vi "Count_Hardness_test.vi"(0 "HS":sgl[](array[numeric]), 1 "TV":sgl[][](array[numeric])) -> (2 "AVG":sgl[](array[numeric]), 3 "HV":sgl[](array[numeric]) format="%#.2g", 4 "REP":sgl[](array[numeric]) format="%#.2g")   [LabVIEW 2019]
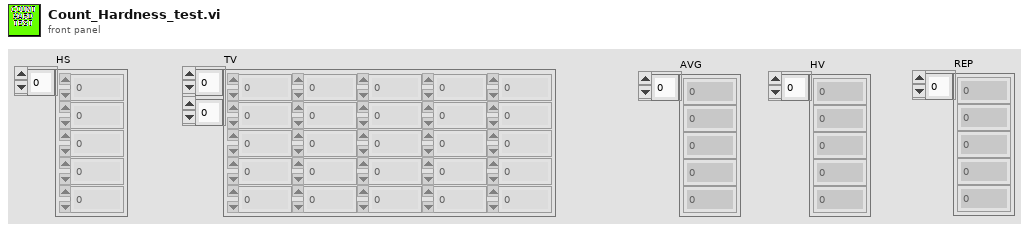
[diagram p1: front panel]
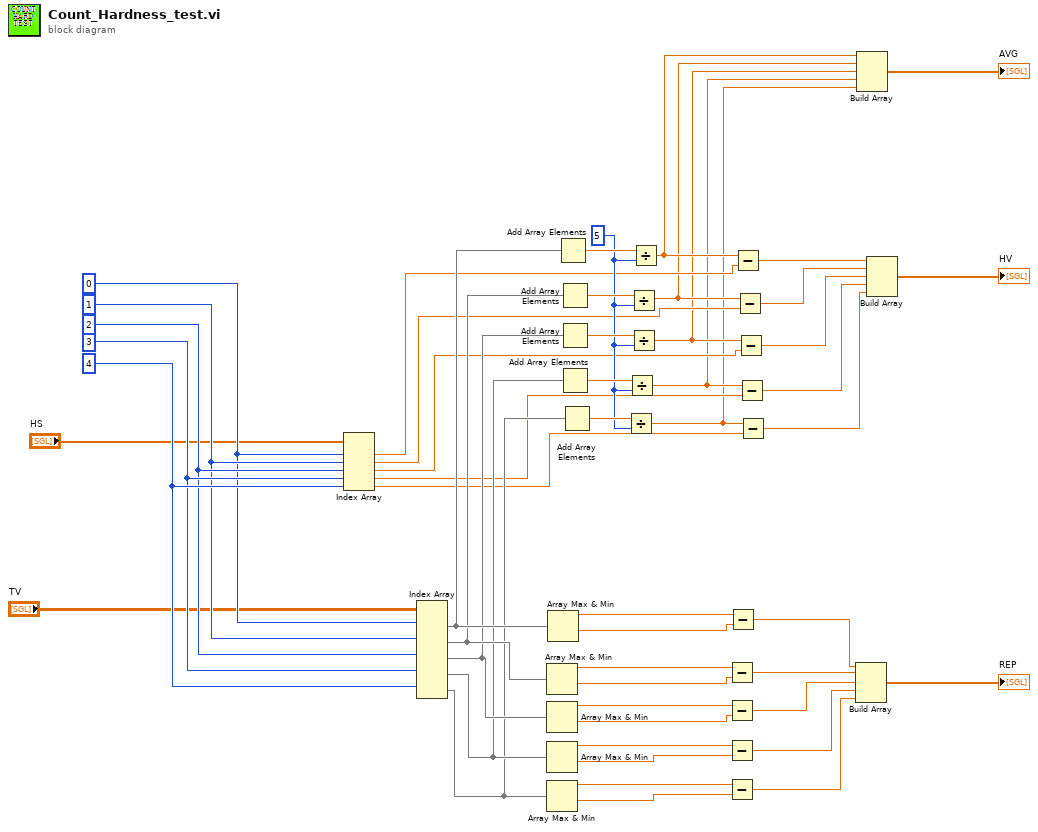
[diagram p0: block diagram]
diagram:
  w34 = 5
  w51 = 4
  w50 = 3
  w49 = 2
  w48 = 1
  w47 = 0
  n1 = Index Array(array="HS", index #1=w47, index #2=w48, index #3=w49, index #4=w50, index #5=w51) -> (element #1=w33:sgl, element #2=w32:sgl, element #3=w31:sgl, element #4=w30:sgl, element #5=w29:sgl)
  n2 = Index Array(array="TV", index (row) #1=w47, index (row) #2=w48, index (row) #3=w49, index (row) #4=w50, index (row) #5=w51) -> (element #1=w44:sgl[], element #2=w43:sgl[], element #3=w42:sgl[], element #4=w41:sgl[], element #5=w40:sgl[])  [unwired: 5 in]
  n3 = Array Max & Min(array=w43) -> (max value=w21:sgl, min value=w20:sgl)  [unwired: 2 out]
  n4 = Array Max & Min(array=w42) -> (max value=w19:sgl, min value=w18:sgl)  [unwired: 2 out]
  n5 = Array Max & Min(array=w41) -> (max value=w17:sgl, min value=w16:sgl)  [unwired: 2 out]
  n6 = Array Max & Min(array=w40) -> (max value=w15:sgl, min value=w14:sgl)  [unwired: 2 out]
  n7 = Array Max & Min(array=w44) -> (max value=w23:sgl, min value=w22:sgl)  [unwired: 2 out]
  n8 = Add Array Elements(numeric array=w44) -> (sum=w39:sgl)
  n9 = Add Array Elements(numeric array=w43) -> (sum=w38:sgl)
  n10 = Add Array Elements(numeric array=w42) -> (sum=w37:sgl)
  n11 = Add Array Elements(numeric array=w41) -> (sum=w36:sgl)
  n12 = Add Array Elements(numeric array=w40) -> (sum=w35:sgl)
  n13 = Divide(x=w35, y=w34) -> (x/y=w2:sgl)
  n14 = Divide(x=w36, y=w34) -> (x/y=w3:sgl)
  n15 = Divide(x=w38, y=w34) -> (x/y=w5:sgl)
  n16 = Divide(x=w37, y=w34) -> (x/y=w4:sgl)
  n17 = Divide(x=w39, y=w34) -> (x/y=w6:sgl)
  n18 = Subtract(x=w21, y=w20) -> (x-y=w12:sgl)
  n19 = Subtract(x=w19, y=w18) -> (x-y=w11:sgl)
  n20 = Subtract(x=w17, y=w16) -> (x-y=w10:sgl)
  n21 = Subtract(x=w15, y=w14) -> (x-y=w9:sgl)
  n22 = Subtract(x=w23, y=w22) -> (x-y=w13:sgl)
  n23 = Subtract(x=w6, y=w33) -> (x-y=w28:sgl)
  n24 = Subtract(x=w5, y=w32) -> (x-y=w27:sgl)
  n25 = Subtract(x=w4, y=w31) -> (x-y=w26:sgl)
  n26 = Subtract(x=w3, y=w30) -> (x-y=w25:sgl)
  n27 = Subtract(x=w2, y=w29) -> (x-y=w24:sgl)
  n28 = Build Array(w13, w12, w11, w10, w9) -> (→"REP":sgl[])
  n29 = Build Array(w6, w5, w4, w3, w2) -> (→"AVG":sgl[])
  n30 = Build Array(w28, w27, w26, w25, w24) -> (→"HV":sgl[])
